vi "Config Format.vi"(6 "Field Width (fixed)":u16(ring) items=["Fixed", "Variable"], 7 "Notation (floating)":u16(ring) items=["Floating", "Scientific", "Engineering"], 8 "error in":errorcluster, 9 "IEEE 488.2 (off)":bool, 10 "Labelling (on)":bool=TRUE, 11 "VISA resource name":refnum<visa-resource-name>) -> (0 "error out":errorcluster, 3 "VISA resource name out":refnum<visa-resource-name>)   [LabVIEW 2017, in "Andeen-Hagerling 2700.lvlib"]
doc: "This VI controls the format and numeric notation of results which are sent to serial or GPIB ports. Front panel results are not affected. Note that default parameter values correspond to the bridge default values and not the values assigned in <b>Default Instrument Setup.vi</b>."
uses:
  Andeen-Hagerling 2700.lvlib
panel:
  # "Format Parameters"
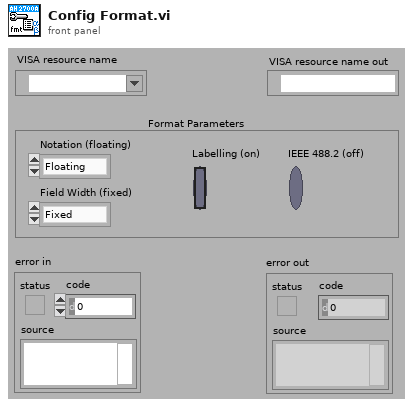
[diagram p1: front panel]
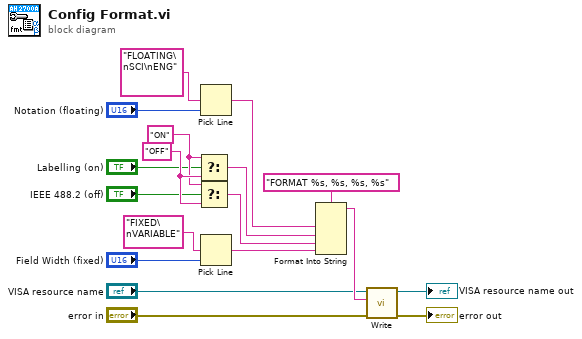
[diagram p0: block diagram]
diagram:
  w18 = "OFF"
  w17 = "ON"
  n1 = Select(t=w17, s="Labelling (on)", f=w18) -> (s? t:f=w8:string)
  n2 = Select(t=w17, s="IEEE 488.2 (off)", f=w18) -> (s? t:f=w7:string)
  n3 = Pick Line(multi-line string="FLOATING\nSCI\nENG", line index="Notation (floating)") -> (output string=w9:string)  [unwired: 1 in]
  n4 = Pick Line(multi-line string="FIXED\nVARIABLE", line index="Field Width (fixed)") -> (output string=w6:string)  [unwired: 1 in]
  n5 = Format Into String(format string="FORMAT %s, %s, %s, %s", w9, w8, w7, w6) -> (resulting string=w16:string)  [unwired: 2 in, 1 out]
  n6 = call "Write.vi"("error in"="error in", "command"=w16, "VISA resource name"="VISA resource name") -> ("error out"=→"error out":errorcluster, "VISA resource name out"=→"VISA resource name out":refnum<visa-resource-name>)  [unwired: 7 in]
